vi "Write Module Init on Error.vi"(7 "Module ID":string, 8 "error in":errorcluster, 10 "Initialize on Error?":bool, 11 "Standard Engine Repo Data in":refnum<class "Standard Engine Configuration.lvclass">) -> (0 "error out":errorcluster, 3 "Standard Engine Repo Data out":refnum<class "Standard Engine Configuration.lvclass">)   [LabVIEW 2013, in "Standard Engine Configuration.lvclass"]
doc: "Specifies the decimation property of a specific module within the engine. A decimation value of 5 will inform the engine to call that module's methods every 5th execution cycle. The offset is a number ranging from 0-'Decimation' and specifies how many iterations pass before the engine calls that module's methods for the first time."
uses:
  Standard Engine Configuration.lvclass
  Standard Engine Configuration.lvclass/Standard Engine Configuration.ctl
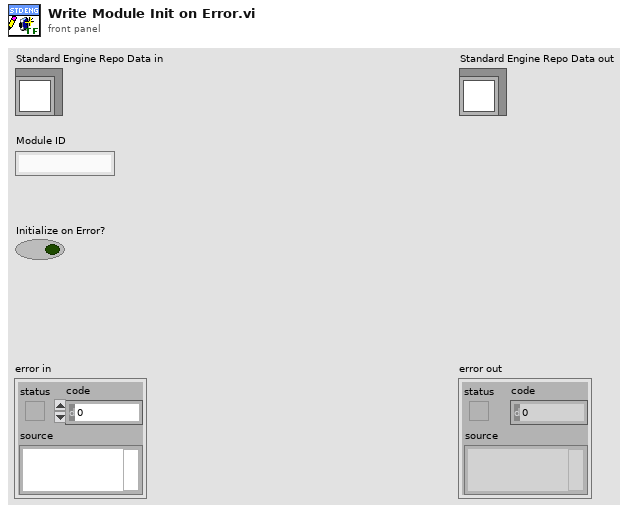
[diagram p1: front panel]
types:
  T1 = typedef "Standard Engine Configuration.lvclass/Module Specific Configuration.ctl" = cluster{"Module ID":string, "Module Decimation":T2, "error tag":string, "error responses":T3, "Initialize on Error?":bool}
  T2 = typedef "Standard Engine Configuration.lvclass/Module Decimation.ctl" = cluster{"Decimation":u16, "Offset":u16, "sort order":i32, "async?":bool}
  T3 = typedef "Standard Engine Configuration.lvclass/error responses.ctl" = cluster{"unknown":T4, "trivial":T4, "critical":T4, "recoverable":T4}
  T4 = typedef "Standard Engine Configuration.lvclass/error options.ctl" = cluster{"clear":bool, "notify":bool, "log":bool, "remove module":bool, "abort engine":bool, "go to safe state":bool, "recover module":bool}
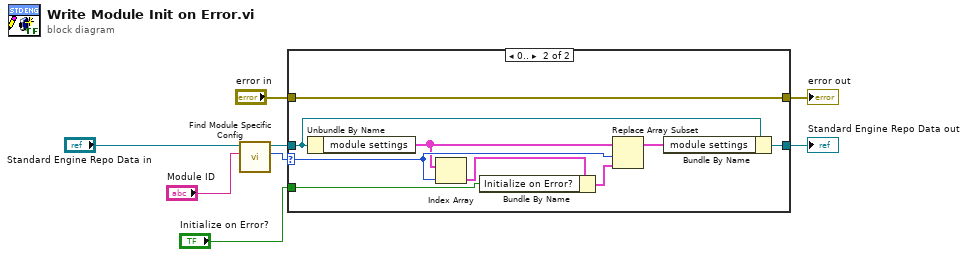
[diagram p0: block diagram]
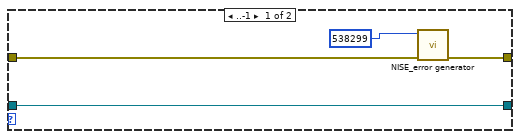
[diagram p2: hidden frame]
diagram:
  n1 = call "Find Module Specific Config.vi"("Module ID"="Module ID", "Standard Engine Repo Data in"="Standard Engine Repo Data in") -> ("Index"=w2:i32, "Standard Engine Repo Data out"=w3:refnum<class "Standard Engine Configuration.lvclass">)  [unwired: 8 in]
  n2 = case shown="0.." w2 {
    selector: w2 -> [_ w21]
    tunnel: w3 -> [w11 w20]
    tunnel: "error in" -> [w12 w17]
    tunnel: [w10 w17] -> w5
    tunnel: [w11 w19] -> w4
    tunnel: "Initialize on Error?" -> [_ w18]
    frame ..-1 {
      n3 = call <vilib>:"NISE_error generator.vi"("error in"=w12, "error code (0)"=538299) -> ("error out"=w10:errorcluster)  [unwired: 7 in]
    }
    frame 0.. {
      n4 = Unbundle By Name(w20) -> ("module settings"=w15:T1[])
      n5 = Index Array(array=w15, index=w21) -> (element=w16:T1)
      n6 = Bundle By Name(cluster=w16, "Initialize on Error?"=w18) -> (w14:T1)
      n7 = Replace Array Subset(array=w15, new element=w14, index=w21) -> (w13:T1[])
      n8 = Bundle By Name(cluster=w20, "module settings"=w13) -> (w19:refnum<class "Standard Engine Configuration.lvclass">)
    }
  }
  "error out" <- w5
  "Standard Engine Repo Data out" <- w4
